vi "Get All Topology Relays.vi"(8 "error in (no error)":errorcluster {"code" format="%.0x"}, 11 "Custom Device Ref in":T1 format="%.0x") -> (0 "error out":errorcluster {"code" format="%.0x"}, 2 "Available Relays":string[](array[string]), 3 "Custom Device Ref out":T1 format="%.0x")   [LabVIEW 2013, in "MUX Custom Device.lvlib"]
uses:
  MUX Custom Device.lvlib
  <vilib>/NI Veristand/Custom Device API/Custom Device Item Ref.ctl
  MUX Global.vi
  <vilib>/NI Veristand/Custom Device API/Get Item Property (String).vi
  <vilib>/NI Veristand/Custom Device API/Custom Device API.lvlib
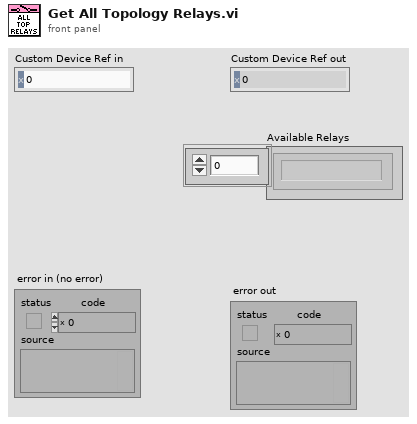
[diagram p1: front panel]
types:
  T1 = typedef "Custom Device API.lvlib/Custom Device Item Ref.ctl" = u64
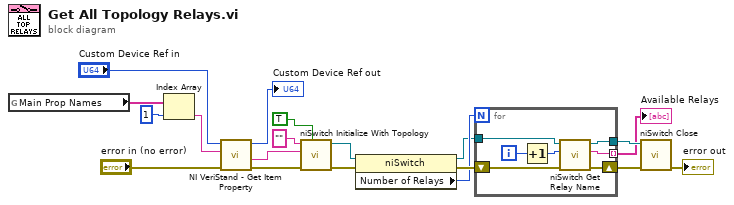
[diagram p0: block diagram]
diagram:
  n1 = global read "MUX Global.vi" "Main Prop Names"() -> (w8:string[])
  n2 = Index Array(array=w8, index=1) -> (element=w6:string)
  n3 = call-poly <vilib>:"NI VeriStand - Get Item Property.vi"("error in (no error)"="error in (no error)", "Property Name"=w6, "Item Ref in"="Custom Device Ref in") -> ("error out"=w3:errorcluster, "Value"=w5:string, "Item Ref out"=→"Custom Device Ref out":T1)  [unwired: 5 in, 1 out]
  n4 = call <instrlib>:"niSwitch Initialize With Topology.vi"("simulate (boolean value)"=TRUE, "error in (no error)"=w3, "topology name"=w5, "resource name"="") -> ("error out"=w14:errorcluster, "instrument handle out"=w15:refnum<k15>)  [unwired: 6 in]
  n5 = property class="niSwitch"(reference=w15, error in=w14) -> (reference out=w11:refnum<k15>, error out=w13:errorcluster, "Number of Relays"=w12:i32)
  n6 = for {
    N: w12 -> [_]
    tunnel: w11 -> [w21]
    tunnel: [w25] -> w9 mode=indexing
    tunnel: [w23] -> w18
    shift-right: [w22] -> w19
    shift-left: w13 -> [w20]
    i -> [w26]
    n7 = Increment(x=w26) -> (x+1=w24:i32)
    n8 = call <instrlib>:"niSwitch Get Relay Name.vi"("error in (no error)"=w20, "index (1)"=w24, "instrument handle"=w21) -> ("error out"=w22:errorcluster, "relay name"=w25:string, "instrument handle out"=w23:refnum<k15>)  [unwired: 6 in]
  }
  "Available Relays" <- w9
  n9 = call <instrlib>:"niSwitch Close.vi"("error in (no error)"=w19, "instrument handle"=w18) -> ("error out"=→"error out":errorcluster)  [unwired: 9 in]
